vi "Manual override - teleop code.vi"(0 "60 Percent":bool, 1 "Increase Speed":bool, 5 "BAck":bool, 6 "Right Limit":bool, 7 "Left Limit":bool, 8 "FIRE!":bool, 9 "Turret Twist":dbl, 10 "Numeric":dbl, 11 "Manual override on?":bool) -> ()   [LabVIEW 2011]
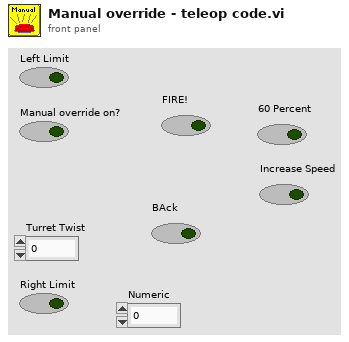
[diagram p1: front panel]
types:
  T1 = typedef "WPI_MotorControlDeviceRef.ctl" = cluster{"DeviceStatus":errorcluster, "Type":enum16{"PWM", "CAN"}, "PWM":cluster{"Digital Module":T2, "PWM Channel":T3, "DeadBand":T4}, "CAN":cluster{"Device Number":u8, "Control Mode":T5, "Semaphore":T6, "Max Vout":dbl}, "Invert":bool, "TransformRef":T7, "InvTransformRef":T7}
  T2 = typedef "FPGA_TypedefDigitalModule.ctl" = enum16{"Digital Module 1", "Digital Module 2"}
  T3 = typedef "FPGA_DIOPWMChannel.ctl" = enum8{"PWM 1", "PWM 2", "PWM 3", "PWM 4", "PWM 5", "PWM 6", "PWM 7", "PWM 8", "PWM 9", "PWM 10", "Invalid"}
  T4 = typedef "WPI_PWMDeadband.ctl" = cluster{"Name":string, "maxPositivePwm":i32, "minPositivePwm":i32, "centerPwm":i32, "maxNegativePwm":i32, "minNegativePwm":i32, "angularRange":u16}
  T5 = typedef "WPI_CANJaguar_ControlMode.ctl" = enum8{"Percent VBus", "Current", "Speed", "Position", "Voltage"}
  T6 = typedef "Semaphore RefNum" = refnum<k1>
  T7 = typedef "WPI_PWMTransform_ConPane.ctl" = refnum<vi>
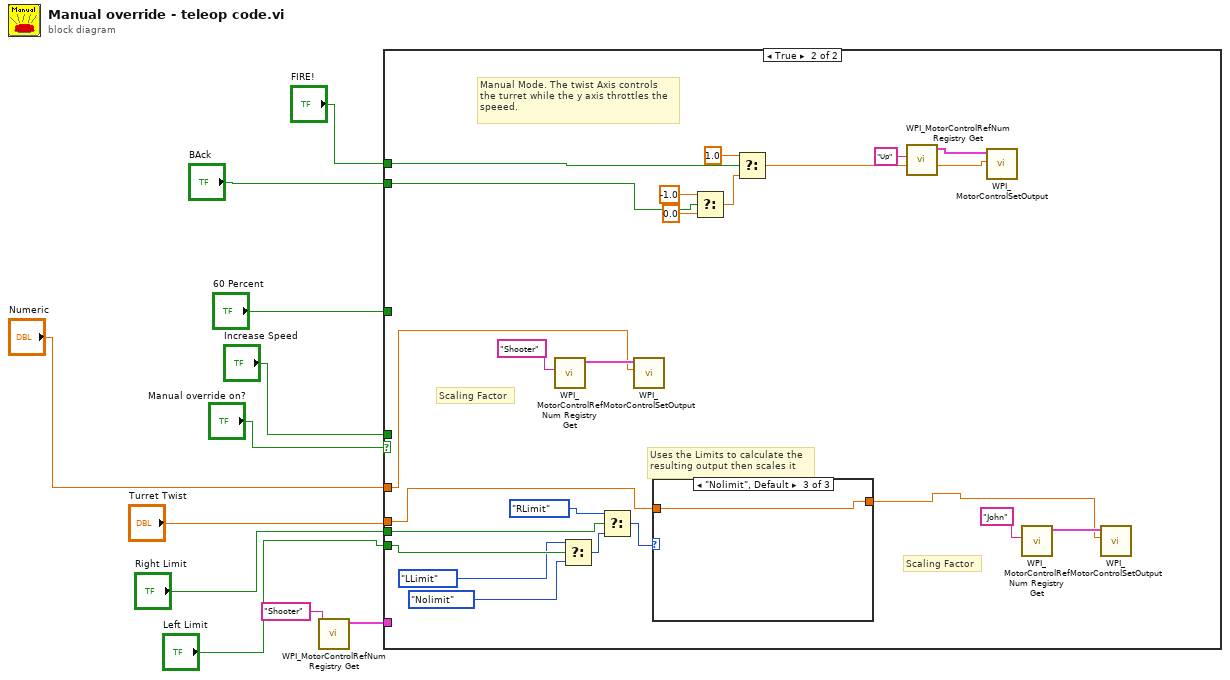
[diagram p0: block diagram]
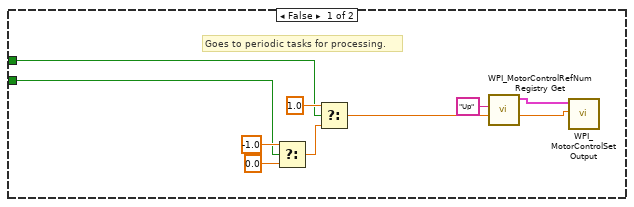
[diagram p2: hidden frame]
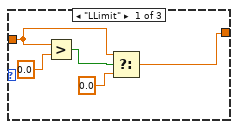
[diagram p3: hidden frame]
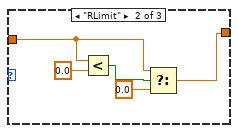
[diagram p4: hidden frame]
diagram:
  n1 = call <vilib>:"WPI_MotorControlRefNum Registry Get.vi"("refnum name"="Shooter") -> ("MotorControlDevRef"=w3:T1)  [unwired: 9 in, 1 out]
  n2 = case shown="True" "Manual override on?" {
    tunnel: "Turret Twist" -> [_ w34]
    tunnel: "Right Limit" -> [_ w37]
    tunnel: "Left Limit" -> [_ w41]
    tunnel: "FIRE!" -> [w13 w31]
    tunnel: "BAck" -> [w12 w25]
    tunnel: "Increase Speed" -> [_ _]
    tunnel: "60 Percent" -> [_ _]
    tunnel: w3 -> [_ _]
    tunnel: "Numeric" -> [_ w21]
    frame False {
      # "Goes to periodic tasks for processing."
      n3 = Select(t=-1.0, s=w12, f=0.0) -> (s? t:f=w18:dbl)
      n4 = Select(t=1.0, s=w13, f=w18) -> (s? t:f=w17:dbl)
      n5 = call <vilib>:"WPI_MotorControlRefNum Registry Get.vi"("refnum name"="Up") -> ("MotorControlDevRef"=w15:T1)  [unwired: 9 in, 1 out]
      n6 = call <vilib>:"WPI_MotorControlSetOutput.vi"("Output"=w17, "MotorControlDevRef"=w15) -> ()  [unwired: 8 in, 2 out]
    }
    frame True {
      # "Scaling Factor"
      # "Uses the Limits to calculate the\nresulting output then scales it"
      # "Scaling Factor"
      # "Manual Mode. The twist Axis controls\nthe turret while the y axis throttles the\nspeeed."
      n7 = call <vilib>:"WPI_MotorControlRefNum Registry Get.vi"("refnum name"="Shooter") -> ("MotorControlDevRef"=w23:T1)  [unwired: 9 in, 1 out]
      n8 = Select(t=enum16{"LLimit", "RLimit", "Nolimit"}."LLimit", s=w41, f=enum16{"LLimit", "RLimit", "Nolimit"}."Nolimit") -> (s? t:f=w38:enum16{"LLimit", "RLimit", "Nolimit"})
      n9 = Select(t=enum16{"LLimit", "RLimit", "Nolimit"}."RLimit", s=w37, f=w38) -> (s? t:f=w35:enum16{"LLimit", "RLimit", "Nolimit"})
      n10 = call <vilib>:"WPI_MotorControlSetOutput.vi"("Output"=w21, "MotorControlDevRef"=w23) -> ()  [unwired: 8 in, 2 out]
      n11 = case shown="\"Nolimit\", Default" w35 {
        tunnel: [w46 w50 w54] -> w28
        tunnel: w34 -> [w45 w49 w54]
        frame "LLimit" {
          n12 = Greater?(x=w45, y=0.0) -> (0:w47:bool)
          n13 = Select(t=w45, s=w47, f=0.0) -> (s? t:f=w46:dbl)
        }
        frame "RLimit" {
          n14 = Less?(x=w49, y=0.0) -> (x < y?=w52:bool)
          n15 = Select(t=w49, s=w52, f=0.0) -> (s? t:f=w50:dbl)
        }
        frame "Nolimit", Default {
        }
      }
      n16 = Select(t=-1.0, s=w25, f=0.0) -> (s? t:f=w27:dbl)
      n17 = Select(t=1.0, s=w31, f=w27) -> (s? t:f=w29:dbl)
      n18 = call <vilib>:"WPI_MotorControlRefNum Registry Get.vi"("refnum name"="Up") -> ("MotorControlDevRef"=w32:T1)  [unwired: 9 in, 1 out]
      n19 = call <vilib>:"WPI_MotorControlSetOutput.vi"("Output"=w29, "MotorControlDevRef"=w32) -> ()  [unwired: 8 in, 2 out]
      n20 = call <vilib>:"WPI_MotorControlRefNum Registry Get.vi"("refnum name"="John") -> ("MotorControlDevRef"=w43:T1)  [unwired: 9 in, 1 out]
      n21 = call <vilib>:"WPI_MotorControlSetOutput.vi"("Output"=w28, "MotorControlDevRef"=w43) -> ()  [unwired: 8 in, 2 out]
    }
  }
